vi "Main UI.vi"(8 "error in (no error)":errorcluster, 11 "SB App in":refnum<class "SB App.lvclass">) -> (0 "error out":errorcluster, 3 "SB App out":refnum<class "SB App.lvclass">)   [LabVIEW 2020, in "SB App.lvlib" / "SB App.lvclass"]
uses:
  SB App.lvclass
  SB App.lvclass/SB App.ctl
  Display Mode.ctl
  SquareBattle/Game/Game.lvclass/Game.ctl
  SquareBattle/Map/Map.lvclass/Map.ctl
  Incoming Events.ctl
  Board Size Update.ctl
  Game Start Data.ctl
  SquareBattle/Team ID.ctl
  Start Position Data.ctl
  SquareBattle/Position.ctl
  0975d5d3-d914-4835-b03b-64ca4af76196.vi
  <vilib>/Utility/High Resolution Relative Seconds.vi
  SB App.lvlib
  SquareBattle/SquareBattle.lvlib
  SquareBattle/Game/Game.lvclass
  Game Config Panel/Game Config Panel.lvclass
  Team Field Panel/Team Field Panel.lvclass
  <vilib>/ptbypt/NI_PtbyPt.lvlib
panel:
  out "Rate":dbl format="%#_2g"
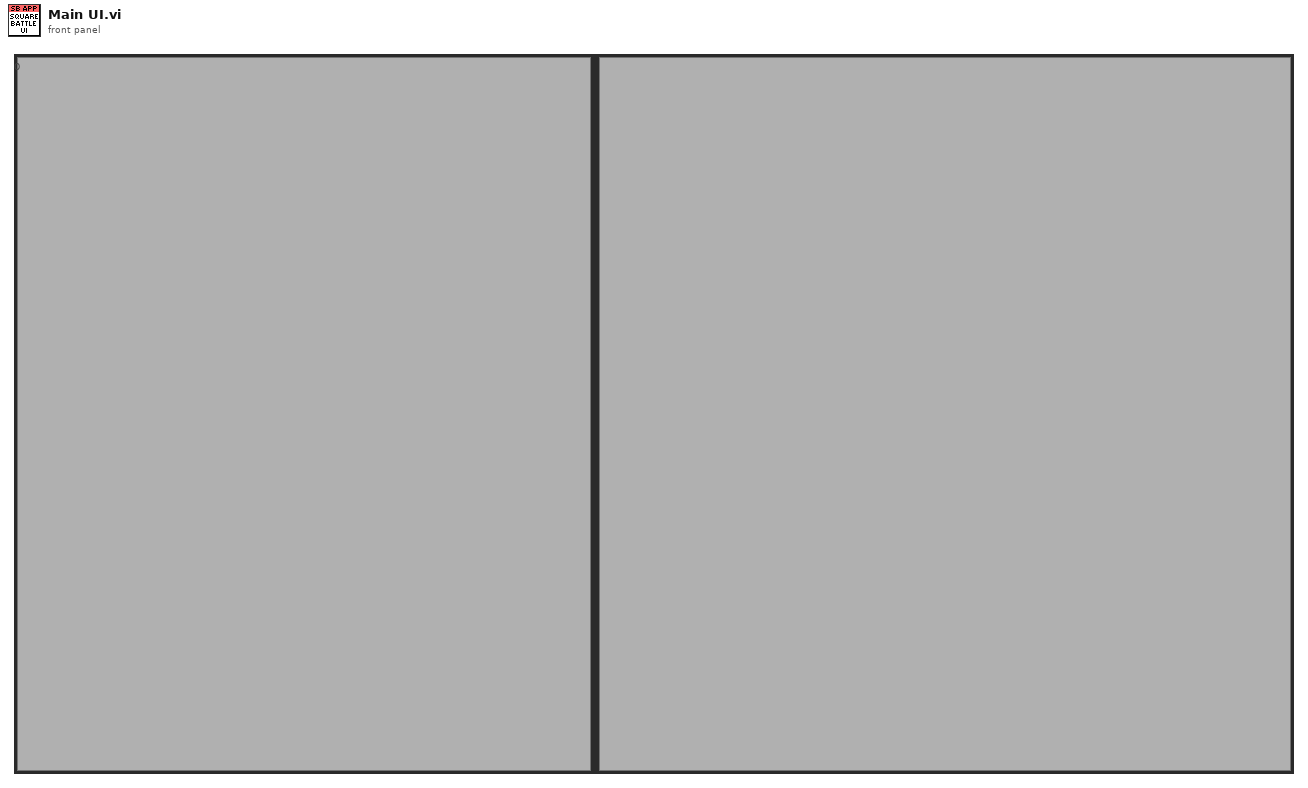
[diagram p1: front panel]
types:
  T1 = enum32{"Invalid", "Standard", "Closed", "Hidden", "Minimized", "Maximized"}
  T2 = typedef "SB App.lvlib/Display Mode.ctl" = enum16{"Config", "Team", "Squares", "Done"}
  T3 = typedef "SB App.lvlib/SB App.lvclass/Incoming Events.ctl" = cluster{"Board Size Update":refnum<user-event>, "Game Start":refnum<user-event>, "Add Team":refnum<user-event>, "Remove Team":refnum<user-event>, "Start Position":refnum<user-event>, "Randomize":refnum<user-event>, "Do Turn":refnum<user-event>, "Stop Battle":refnum<user-event>, "Rep Rounds":refnum<user-event>, "Config Video":refnum<user-event>}
  T4 = typedef "SquareBattle.lvlib/Team ID.ctl" = u32
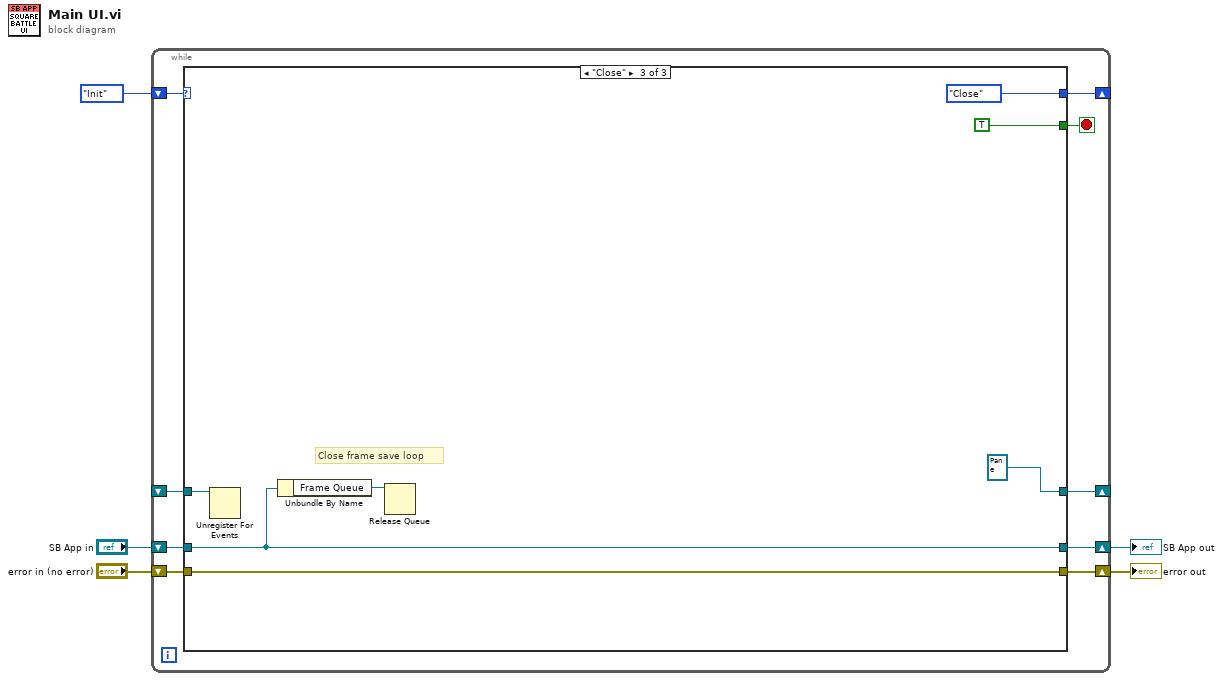
[diagram p0: block diagram]
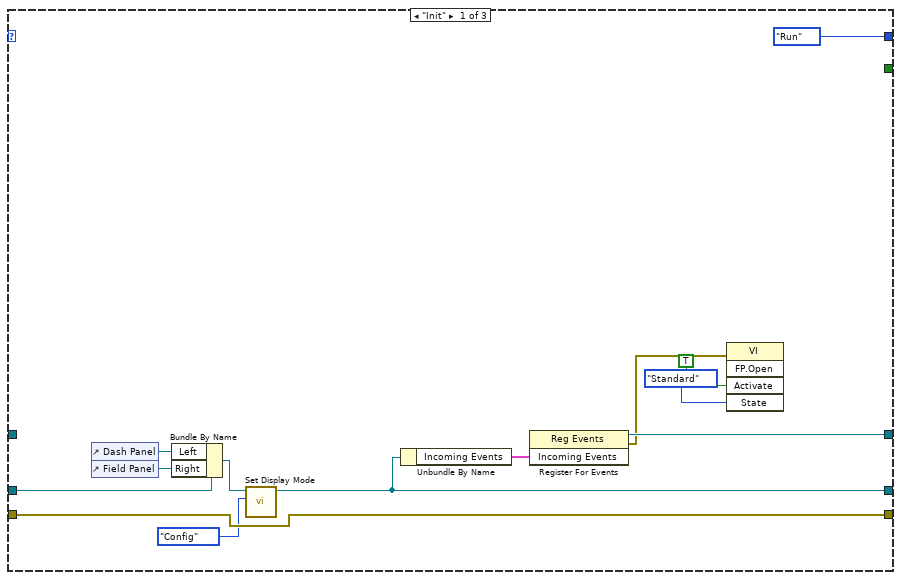
[diagram p2: hidden frame]
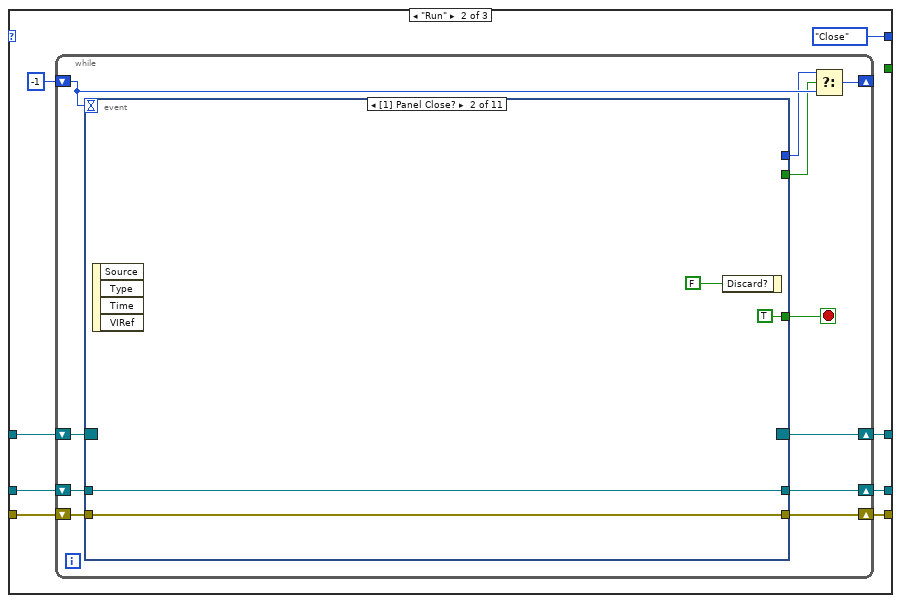
[diagram p3: hidden frame]
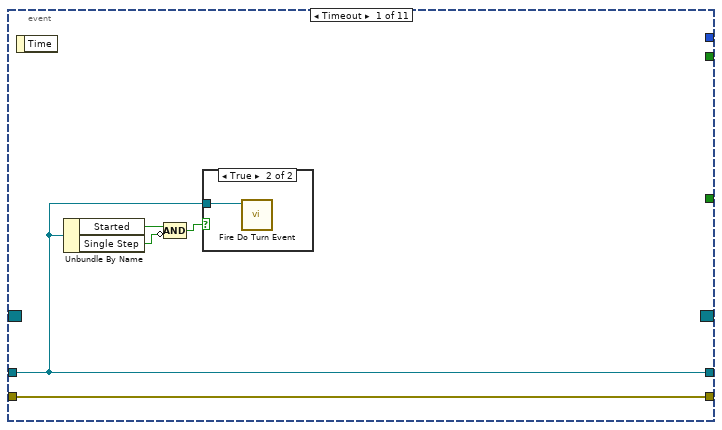
[diagram p4: hidden frame]
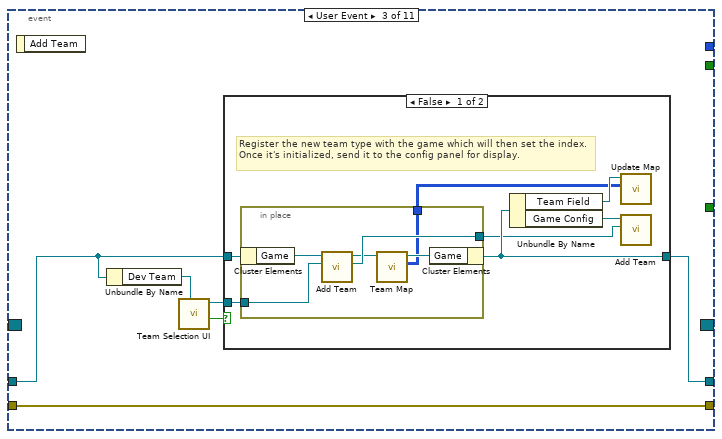
[diagram p6: hidden frame]
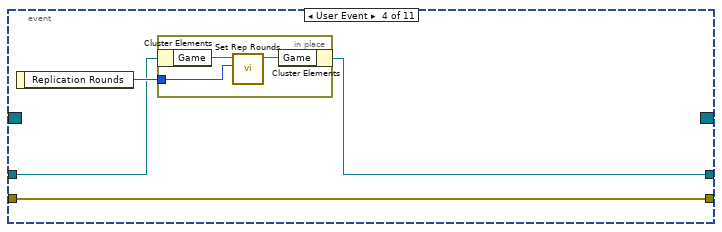
[diagram p8: hidden frame]
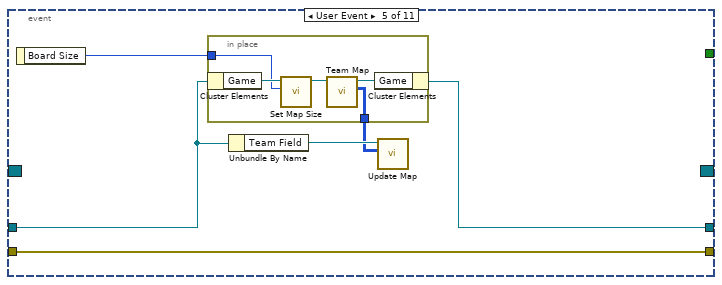
[diagram p9: hidden frame]
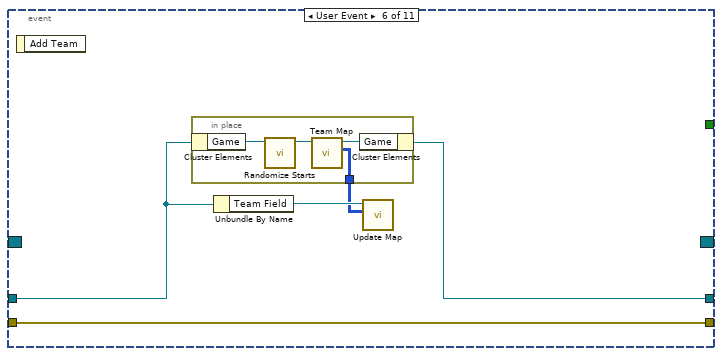
[diagram p10: hidden frame]
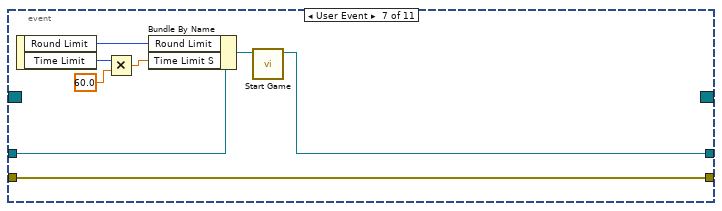
[diagram p11: hidden frame]
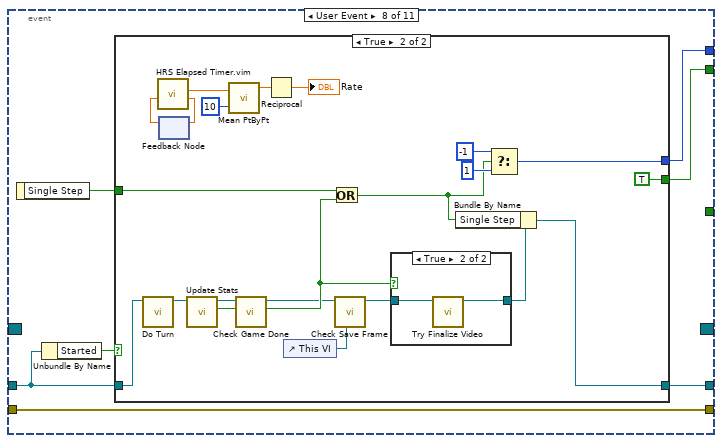
[diagram p12: hidden frame]
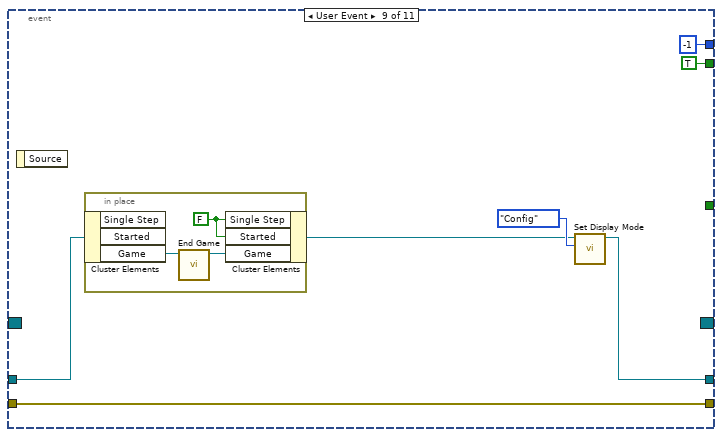
[diagram p15: hidden frame]
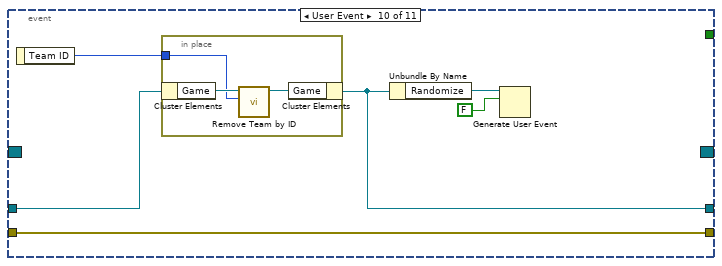
[diagram p16: hidden frame]
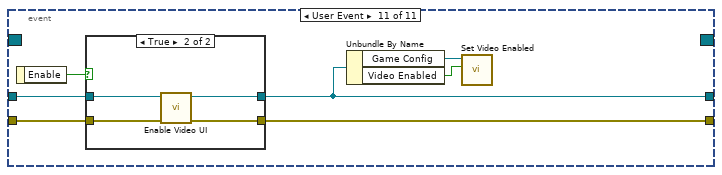
[diagram p17: hidden frame]
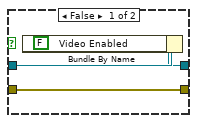
[diagram p18: hidden frame]
diagram:
  n1 = while {
    shift-right: [w13] -> _
    shift-left: enum16{"Init", "Run", "Close"}."Init" ("Basic UI State") -> [w14]
    shift-right: [w8] -> w3
    shift-left: "SB App in" -> [w12]
    shift-right: [w9] -> w2
    shift-left: "error in (no error)" -> [w11]
    shift-right: [w7] -> _
    shift-left: _ -> [w6]
    stop <- w10 stop-if-true
    n2 = case shown="\"Close\"" w14 {
      tunnel: [enum16{"Init", "Run", "Close"}."Run" ("Basic UI State") enum16{"Init", "Run", "Close"}."Close" ("Basic UI State") enum16{"Init", "Run", "Close"}."Close" ("Basic UI State")] -> w13
      tunnel: w12 -> [w26 w34 w180]
      tunnel: w11 -> [w20 w33 w183]
      tunnel: [_ _ TRUE] -> w10
      tunnel: [w20 w31 w183] -> w9
      tunnel: [w18 w32 w180] -> w8
      tunnel: [w22 w29 refnum<event-registration> refnum ("Event Registration Refnum")] -> w7
      tunnel: w6 -> [_ w30 w182]
      frame "Init" {
        n3 = control-ref of="Dash Panel"() -> (w25:refnum<vi>)
        n4 = control-ref of="Field Panel"() -> (w24:refnum<vi>)
        n5 = Bundle By Name(cluster=w26, "Left"=w25, "Right"=w24) -> (w19:refnum<class "SB App.lvclass">)
        n6 = call "Set Display Mode.vi"("Display Mode"=Display_Mode."Config", "SB App in"=w19) -> ("SB App out"=w18:refnum<class "SB App.lvclass">)  [unwired: 9 in]
        n7 = Unbundle By Name(w18) -> ("Incoming Events"=w23:T3)
        n8 = register-events(w23) -> (reference out=w22:refnum<event-registration>, error out=w21:errorcluster)  [unwired: 2 in]
        n9 = invoke class="VI" method="FP.Open"(error in=w21, "Activate"=TRUE ("Activate?"), "State"=T1."Standard") -> ()  [unwired: 2 in, 5 out]
      }
      frame "Run" {
        n10 = while {
          shift-right: [w43] -> w32
          shift-left: w34 -> [w46]
          shift-right: [w42] -> w31
          shift-left: w33 -> [w45]
          shift-right: [w41] -> w29
          shift-left: w30 -> [w36]
          shift-right: [w40] -> _
          shift-left: -1 -> [w39]
          stop <- w44 stop-if-true
          n11 = event shown="[1] Panel Close?" {
            selector: w36 -> [_ _ _ _ _ _ _ _ _ _ _]
            dyn-events: [_ _ _ _ _ _ _ _ _ _ _] -> w41
            timeout: w39 -> [_ _ _ _ _ _ _ _ _ _ _]
            tunnel: w46 -> [w50 w56 w58 w78 w86 w96 w108 w116 w148 w159 w169]
            tunnel: w45 -> [w51 w55 w62 w80 w89 w99 w111 w118 w151 w160 w168]
            tunnel: [_ TRUE ("Discard?") _ _ _ _ _ _ _ _ _] -> w44
            tunnel: [w50 w56 w59 w77 w87 w95 w104 w112 w150 w157 w166] -> w43
            tunnel: [w51 w55 w62 w80 w89 w99 w111 w118 w151 w160 w167] -> w42
            tunnel: [_ _ _ _ _ _ _ w114 TRUE _ _] -> w38
            tunnel: [_ _ _ _ _ _ _ w113 -1 ("f") _ _] -> w37
            event Timeout {
              n12 = event-data() -> ()  [unwired: 1 in, 1 out]
              n13 = Unbundle By Name(w50) -> ("Started"=w49:bool, "Single Step"=w48:bool)
              n14 = Compound Arithmetic op=AND(w49, invert w48) -> (w47:bool)
              n15 = case shown="True" w47 {
                tunnel: w50 -> [_ w52]
                frame False {
                }
                frame True {
                  n16 = call "Fire Do Turn Event.vi"("SB App in"=w52) -> ()  [unwired: 10 in, 1 out]
                }
              }
            }
            event Panel Close? {
              n17 = event-data() -> ()  [unwired: 1 in, 4 out]
              n18 = event-data("Discard?"=FALSE) -> ()  [unwired: 1 in, 1 out]
            }
            event User Event {
              n19 = event-data() -> ()  [unwired: 1 in, 1 out]
              n20 = Unbundle By Name(w58) -> ("Dev Team"=w57:refnum<class "Team.lvclass">)
              n21 = call "Team Selection UI.vi"("Dev Team"=w57) -> ("Cancelled"=w60:bool, "Team"=w61:refnum<class "Team.lvclass">)  [unwired: 9 in]
              n22 = case shown="False" w60 {
                tunnel: w58 -> [w69 w76]
                tunnel: w61 -> [w68 _]
                tunnel: [w67 w76] -> w59
                frame False {
                  # "Register the new team type with the game which will then set the index. Once it's initialized, send it to the config panel for display."
                  n23 = in-place {
                    in-place-border: w68 -> [w74]
                    in-place-border: [w73] -> w65
                    in-place-border: [w70] -> w63
                    n24 = in-place-cluster #1(w69) -> ("Game"=w75:refnum<class "Game.lvclass">)
                    n25 = call "Add Team.vi"("Team Type"=w74, "Game in"=w75) -> ("Team"=w73:refnum<class "Team.lvclass">, "Game out"=w72:refnum<class "Game.lvclass">)  [unwired: 7 in, 1 out]
                    n26 = call "Team Map.vi"("Game in"=w72) -> ("Team Map"=w70:i32[][], "Game out"=w71:refnum<class "Game.lvclass">)  [unwired: 9 in]
                    n27 = in-place-cluster #1("Game"=w71) -> (w67:refnum<class "SB App.lvclass">)
                  }
                  n28 = Unbundle By Name(w67) -> ("Team Field"=w64:refnum<class "Team Field Panel.lvclass">, "Game Config"=w66:refnum<class "Game Config Panel.lvclass">)
                  n29 = call "Update Map.vi"("Team Map"=w63, "Team Field Panel in"=w64) -> ()  [unwired: 8 in, 2 out]
                  n30 = call "Add Team.vi"("Team"=w65, "Game Config Panel in"=w66) -> ()  [unwired: 8 in, 2 out]
                }
                frame True {
                  # "User cancelled selection, don't need to do anything."
                }
              }
            }
            event User Event {
              n31 = event-data() -> ("Replication Rounds"=w79:u32)  [unwired: 1 in]
              n32 = in-place {
                in-place-border: w79 -> [w82]
                n33 = in-place-cluster #2(w78) -> ("Game"=w83:refnum<class "Game.lvclass">)
                n34 = call "Set Rep Rounds.vi"("Rep Rounds"=w82, "Game in"=w83) -> ("Game out"=w81:refnum<class "Game.lvclass">)  [unwired: 8 in, 1 out]
                n35 = in-place-cluster #2("Game"=w81) -> (w77:refnum<class "SB App.lvclass">)
              }
            }
            event User Event {
              n36 = event-data() -> ("Board Size"=w88:i32)  [unwired: 1 in]
              n37 = in-place {
                in-place-border: w88 -> [w93]
                in-place-border: [w91] -> w84
                n38 = in-place-cluster #3(w86) -> ("Game"=w94:refnum<class "Game.lvclass">)
                n39 = call "Set Map Size.vi"("Map Size"=w93, "Game in"=w94) -> ("Game out"=w90:refnum<class "Game.lvclass">)  [unwired: 8 in, 1 out]
                n40 = call "Team Map.vi"("Game in"=w90) -> ("Team Map"=w91:i32[][], "Game out"=w92:refnum<class "Game.lvclass">)  [unwired: 9 in]
                n41 = in-place-cluster #3("Game"=w92) -> (w87:refnum<class "SB App.lvclass">)
              }
              n42 = Unbundle By Name(w86) -> ("Team Field"=w85:refnum<class "Team Field Panel.lvclass">)
              n43 = call "Update Map.vi"("Team Map"=w84, "Team Field Panel in"=w85) -> ()  [unwired: 8 in, 2 out]
            }
            event User Event {
              n44 = event-data() -> ()  [unwired: 1 in, 1 out]
              n45 = in-place {
                in-place-border: [w102] -> w97
                n46 = in-place-cluster #4(w96) -> ("Game"=w101:refnum<class "Game.lvclass">)
                n47 = call "Randomize Starts.vi"("Game in"=w101) -> ("Game out"=w100:refnum<class "Game.lvclass">)  [unwired: 9 in, 1 out]
                n48 = call "Team Map.vi"("Game in"=w100) -> ("Team Map"=w102:i32[][], "Game out"=w103:refnum<class "Game.lvclass">)  [unwired: 9 in]
                n49 = in-place-cluster #4("Game"=w103) -> (w95:refnum<class "SB App.lvclass">)
              }
              n50 = Unbundle By Name(w96) -> ("Team Field"=w98:refnum<class "Team Field Panel.lvclass">)
              n51 = call "Update Map.vi"("Team Map"=w97, "Team Field Panel in"=w98) -> ()  [unwired: 8 in, 2 out]
            }
            event User Event {
              n52 = event-data() -> ("Round Limit"=w106:u32, "Time Limit"=w105:i32)  [unwired: 1 in]
              n53 = Multiply(x=w105, y=60.0) -> (x*y=w109:dbl)
              n54 = Bundle By Name(cluster=w108, "Round Limit"=w106, "Time Limit S"=w109) -> (w107:refnum<class "SB App.lvclass">)
              n55 = call "Start Game.vi"("SB App in"=w107) -> ("SB App out"=w104:refnum<class "SB App.lvclass">)  [unwired: 10 in]
            }
            event User Event {
              n56 = event-data() -> ("Single Step"=w117:bool)  [unwired: 1 in]
              n57 = Unbundle By Name(w116) -> ("Started"=w115:bool)
              n58 = case shown="True" w115 {
                tunnel: w117 -> [_ w137]
                tunnel: w116 -> [w119 w129]
                tunnel: [_ TRUE] -> w114
                tunnel: [_ w139] -> w113
                tunnel: [w119 w128] -> w112
                frame False {
                }
                frame True {
                  n59 = call "Do Turn.vi"("SB App in"=w129) -> ("SB App out"=w130:refnum<class "SB App.lvclass">)  [unwired: 10 in]
                  n60 = feedback #5() -> (w136:dbl)  [unwired: 1 in]
                  n61 = call "HRS Elapsed Timer.vim"("HRS In"=w136) -> ("HRS"=w135:dbl, "Elapsed"=w134:dbl)  [unwired: 7 in, 2 out]
                  n62 = feedback-in #5(w135) -> ()
                  n63 = call "Update Stats.vi"("SB App in"=w130) -> ("Won?"=w122:bool, "SB App out"=w123:refnum<class "SB App.lvclass">)  [unwired: 8 in, 1 out]
                  n64 = call <vilib>:"Mean PtByPt.vi"("x"=w134, "sample length"=10) -> ("mean"=w132:dbl)  [unwired: 2 in, 1 out]
                  n65 = call "Check Game Done.vi"("Won"=w122, "SB App in"=w123) -> ("Done?"=w121:bool, "SB App out"=w120:refnum<class "SB App.lvclass">)  [unwired: 7 in, 1 out]
                  n66 = Reciprocal(x=w132) -> (1/x=→"Rate":dbl)
                  n67 = control-ref of="This VI"() -> (w124:refnum<vi>)
                  n68 = Or(x=w137, y=w121) -> (x .or. y?=w127:bool)
                  n69 = call "Check Save Frame.vi"("Main UI"=w124, "SB App in"=w120) -> ("SB App out"=w126:refnum<class "SB App.lvclass">)  [unwired: 8 in, 1 out]
                  n70 = case shown="True" w121 {
                    tunnel: w126 -> [w142 w144]
                    tunnel: [w142 w143] -> w125
                    frame False {
                    }
                    frame True {
                      n71 = call "Try Finalize Video.vi"("SB App in"=w144) -> ("SB App out"=w143:refnum<class "SB App.lvclass">)  [unwired: 9 in, 1 out]
                    }
                  }
                  n72 = Bundle By Name(cluster=w125, "Single Step"=w127) -> (w128:refnum<class "SB App.lvclass">)
                  n73 = Select(t=-1, s=w127, f=1) -> (s? t:f=w139:i32)
                }
              }
            }
            event User Event {
              n74 = event-data() -> ()  [unwired: 1 in, 1 out]
              n75 = in-place {
                w154 = FALSE ("Single Step")
                n76 = in-place-cluster #6(w148) -> ("Game"=w153:refnum<class "Game.lvclass">)  [unwired: 2 out]
                n77 = call "End Game.vi"("Game in"=w153) -> ("Game out"=w152:refnum<class "Game.lvclass">)  [unwired: 9 in, 1 out]
                n78 = in-place-cluster #6("Single Step"=w154, "Started"=w154, "Game"=w152) -> (w147:refnum<class "SB App.lvclass">)
              }
              n79 = call "Set Display Mode.vi"("Display Mode"=Display_Mode."Config", "SB App in"=w147) -> ("SB App out"=w150:refnum<class "SB App.lvclass">)  [unwired: 9 in]
            }
            event User Event {
              n80 = event-data() -> ("Team ID"=w158:T4)  [unwired: 1 in]
              n81 = in-place {
                in-place-border: w158 -> [w162]
                n82 = in-place-cluster #7(w159) -> ("Game"=w163:refnum<class "Game.lvclass">)
                n83 = call "Remove Team by ID.vi"("Team ID"=w162, "Game in"=w163) -> ("Game out"=w161:refnum<class "Game.lvclass">)  [unwired: 8 in, 1 out]
                n84 = in-place-cluster #7("Game"=w161) -> (w157:refnum<class "SB App.lvclass">)
              }
              n85 = Unbundle By Name(w157) -> ("Randomize"=w156:refnum<user-event>)
              n86 = Generate User Event(user event=w156, event data cluster=FALSE ("event data")) -> ()  [unwired: 2 in, 2 out]
            }
            event User Event {
              n87 = event-data() -> ("Enable"=w170:bool)  [unwired: 1 in]
              n88 = case shown="True" w170 {
                tunnel: w169 -> [w174 w178]
                tunnel: w168 -> [w171 w177]
                tunnel: [w172 w176] -> w166
                tunnel: [w171 w175] -> w167
                frame False {
                  n89 = Bundle By Name(cluster=w174, "Video Enabled"=FALSE) -> (w172:refnum<class "SB App.lvclass">)
                }
                frame True {
                  n90 = call "Enable Video UI.vi"("error in (no error)"=w177, "SB App in"=w178) -> ("error out"=w175:errorcluster, "SB App out"=w176:refnum<class "SB App.lvclass">)  [unwired: 8 in]
                }
              }
              n91 = Unbundle By Name(w166) -> ("Game Config"=w165:refnum<class "Game Config Panel.lvclass">, "Video Enabled"=w164:bool)
              n92 = call "Set Video Enabled.vi"("Video Enabled"=w164, "Game Config Panel in"=w165) -> ()  [unwired: 8 in, 2 out]
            }
          }
          n93 = Select(t=w37, s=w38, f=w39) -> (s? t:f=w40:i32)
        }
      }
      frame "Close" {
        # "Close frame save loop"
        n94 = Unregister For Events(event registration refnum=w182) -> ()  [unwired: 1 in, 1 out]
        n95 = Unbundle By Name(w180) -> ("Frame Queue"=w179:refnum<queue>)
        n96 = Release Queue(queue=w179) -> ()  [unwired: 2 in, 3 out]
      }
    }
  }
  "error out" <- w2
  "SB App out" <- w3
